vi "Write SystemStatus Event.vi"(8 "error in":errorcluster, 10 "SystemStatus Event":refnum<user-event>, 11 "Engine in":refnum<class "Engine.lvclass">) -> (0 "error out":errorcluster, 3 "Engine out":refnum<class "Engine.lvclass">)   [LabVIEW 2019, in "Engine.lvlib" / "Engine.lvclass"]
uses:
  Project/Engine.lvclass
  Custom Controls/System Status.ctl
  Project/Engine.lvclass/Engine.ctl
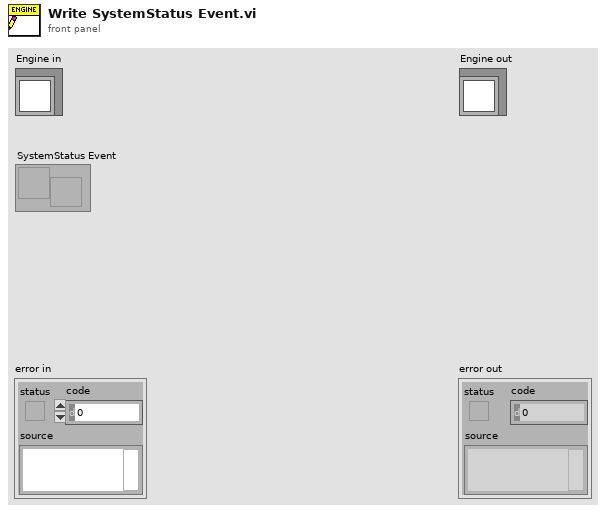
[diagram p1: front panel]
types:
  T1 = typedef "Engine.lvlib/Engine.lvclass/System Status.ctl" = enum16{"Logged Off", "UUT_Info_Missing", "Idle", "Error", "Warning", "Loading", "Config", "Manual", "Automation", "Report_View", "Previous"}
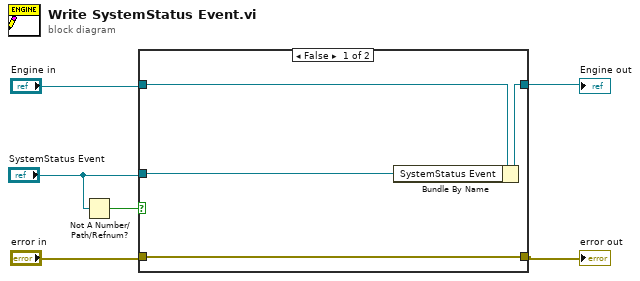
[diagram p0: block diagram]
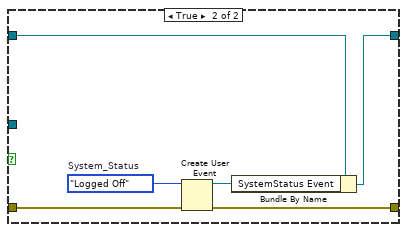
[diagram p2: hidden frame]
diagram:
  n1 = Not A Number/Path/Refnum?(number/path/refnum="SystemStatus Event") -> (NaN/Path/Refnum?=w4:bool)
  n2 = case shown="False" w4 {
    tunnel: [w7 w14] -> w3
    tunnel: [w9 w13] -> w2
    tunnel: "Engine in" -> [w10 w16]
    tunnel: "SystemStatus Event" -> [w8 _]
    tunnel: "error in" -> [w7 w15]
    frame False {
      n3 = Bundle By Name(cluster=w10, "SystemStatus Event"=w8) -> (w9:refnum<class "Engine.lvclass">)
    }
    frame True {
      w12 = System_Status."Logged Off"  # System_Status
      n4 = Create User Event(user event datatype=w12, error in=w15) -> (user event=w11:refnum<user-event>, error out=w14:errorcluster)
      n5 = Bundle By Name(cluster=w16, "SystemStatus Event"=w11) -> (w13:refnum<class "Engine.lvclass">)
    }
  }
  "error out" <- w3
  "Engine out" <- w2
